vi "WSVCAP SHL FPGA LL Configuration File Handler.vi"(0 "Object Cluster In":T3={"Settings"={"FPGA Resource Name"="", "I2C Slave Address"=20, "I2C Clock Rate (Hz)"=50000.0, "SPI Clock Rate (Hz)"=50000.0, "RFFE Slave Address"=20, "RFFE Clock Rate (Hz)"=50000.0, "Simulate FPGA"=TRUE}, "FPGA Resource"="", "Online"=FALSE, "I2C Wait Ticks"=0, "SPI Wait Ticks"=0, "RFFE Wait Ticks"=0} {"Settings"."RFFE Clock Rate (Hz)" format="%.0f Hz"; "Settings"."RFFE Slave Address" format="0x%02x"; "Settings"."I2C Clock Rate (Hz)" format="%.0f Hz"; "Settings"."SPI Clock Rate (Hz)" format="%.0f Hz"; "Settings"."I2C Slave Address" format="0x%02x"}, 1 "Copy Path":path, 2 "System Cfg":T2={"Configuration File Path"=path "inifiles/System Configuration.ini"}, 7 "Copy Tag":string, 11 "Error In (no error)":errorcluster, 12 "Keys (Empty:All)":T1[](array[typedef]), 13 "Operation":T5) -> (4 "Object Cluster Out":T3={"Settings"={"FPGA Resource Name"="", "I2C Slave Address"=20, "I2C Clock Rate (Hz)"=50000.0, "SPI Clock Rate (Hz)"=50000.0, "RFFE Slave Address"=20, "RFFE Clock Rate (Hz)"=50000.0, "Simulate FPGA"=TRUE}, "FPGA Resource"="", "Online"=FALSE, "I2C Wait Ticks"=0, "SPI Wait Ticks"=0, "RFFE Wait Ticks"=0} {"Settings"."RFFE Clock Rate (Hz)" format="%.0f Hz"; "Settings"."RFFE Slave Address" format="0x%02x"; "Settings"."I2C Clock Rate (Hz)" format="%.0f Hz"; "Settings"."SPI Clock Rate (Hz)" format="%.0f Hz"; "Settings"."I2C Slave Address" format="0x%02x"}, 8 "Cancelled":bool, 15 "Error Out":errorcluster)   [LabVIEW 2012]
uses:
  Type Defs/WSVCAP SHL Core System Cluster.ctl
  Type Defs/WSVCAP SHL I2C Settings Cluster.ctl
  user.lib/Configuration Files/Type Defs/CFG File Operation Enum.ctl
  Type Defs/WSVCAP SHL Configuration Items Enum.ctl
  user.lib/Configuration Files/Type Defs/CFG System Configuration Settings Cluster.ctl
panel:
  in  "Config Enum":T1=enum."Settings::Simulate FPGA"
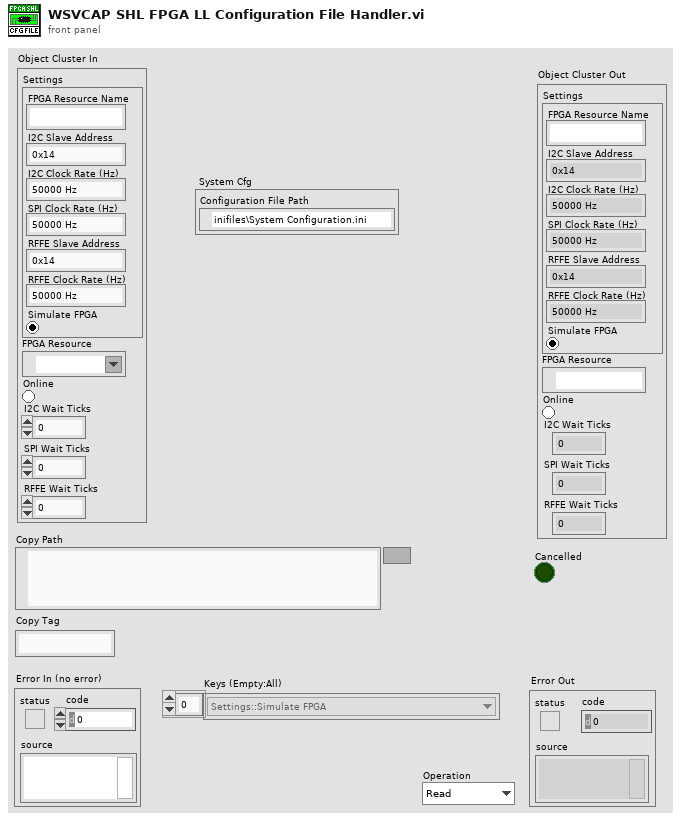
[diagram p1: front panel]
types:
  T1 = typedef "WSVCAP SHL Configuration Items Enum.ctl" = enum16{"Settings::FPGA Resource Name", "Settings::I2C Slave Address", "Settings::I2C Clock Rate (Hz)", "Settings::SPI Clock Rate (Hz)", "Settings::RFFE Slave Address", "Settings::RFFE Clock Rate (Hz)", "Settings::Simulate FPGA"}
  T2 = typedef "CFG System Configuration Settings Cluster.ctl" = cluster{"Configuration File Path":path}
  T3 = typedef "WSVCAP SHL Core System Cluster.ctl" = cluster{"Settings":T4, "FPGA Resource":tag, "Online":bool, "I2C Wait Ticks":u32, "SPI Wait Ticks":u32, "RFFE Wait Ticks":u32}
  T4 = typedef "WSVCAP SHL I2C Settings Cluster.ctl" = cluster{"FPGA Resource Name":string, "I2C Slave Address":u8, "I2C Clock Rate (Hz)":dbl, "SPI Clock Rate (Hz)":dbl, "RFFE Slave Address":u8, "RFFE Clock Rate (Hz)":dbl, "Simulate FPGA":bool}
  T5 = typedef "CFG File Operation Enum.ctl" = enum16{"Read", "Write", "Copy", "Edit"}
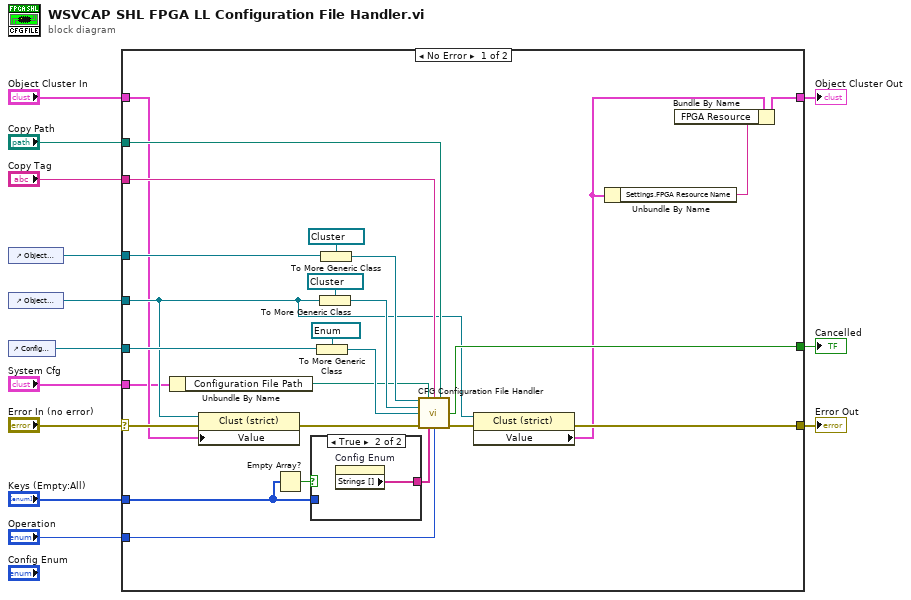
[diagram p0: block diagram]
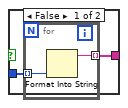
[diagram p2: hidden frame]
diagram:
  n1 = control-ref of="Object Cluster In"() -> (w3:refnum<vi>)
  n2 = control-ref of="Object Cluster Out"() -> (w1:refnum<vi>)
  n3 = control-ref of="Config Enum"() -> (w2:refnum<vi>)
  n4 = case shown="No Error" "Error In (no error)" {
    selector: "Error In (no error)" -> [w22 w46]
    tunnel: [w35 w46] -> w11
    tunnel: "Copy Path" -> [w37 _]
    tunnel: "Copy Tag" -> [w38 _]
    tunnel: "Operation" -> [w39 _]
    tunnel: [w15 w45] -> w7
    tunnel: "Object Cluster In" -> [w19 w45]
    tunnel: w3 -> [w31 _]
    tunnel: w1 -> [w20 _]
    tunnel: w2 -> [w30 _]
    tunnel: "Keys (Empty:All)" -> [w26 _]
    tunnel: [w23 _] -> w5
    tunnel: "System Cfg" -> [w18 _]
    frame No Error {
      n5 = Unbundle By Name(w18) -> ("Configuration File Path"=w17:path)
      n6 = property class="Clust (strict)"(reference=w20, error in=w22, "Value"=w19) -> (error out=w21:errorcluster)  [unwired: 1 out]
      n7 = Empty Array?(array=w26) -> (empty?=w25:bool)
      n8 = case shown="True" w25 {
        tunnel: w26 -> [w41 _]
        tunnel: [w40 w44] -> w24
        frame False {
          n9 = for {
            tunnel: w41 -> [w43] mode=indexing
            tunnel: [w42] -> w40 mode=indexing
            n10 = Format Into String(w43) -> (resulting string=w42:string)  [unwired: 3 in, 1 out]
          }
        }
        frame True {
          n11 = property on="Config Enum" class="Enum (strict)"() -> ("Strings []"=w44:string[])  [unwired: 2 in, 2 out]
        }
      }
      n12 = To More Generic Class(target class=refnum<vi> refnum ("Enum Ref"), reference=w30) -> (generic class reference=w27:refnum<vi>)
      n13 = To More Generic Class(target class=refnum<vi> refnum ("Cluster Ref"), reference=w20) -> (generic class reference=w28:refnum<vi>)
      n14 = To More Generic Class(target class=refnum<vi> refnum ("Cluster Ref"), reference=w31) -> (generic class reference=w29:refnum<vi>)
      n15 = call "CFG Configuration File Handler.vi"("Cluster In Ref"=w29, "System Configuration File"=w17, "Copy Tag"=w38, "Copy Path"=w37, "Cluster Out Ref"=w28, "Enum Ref"=w27, "Error In (no error)"=w21, "Keys (Empty:All)"=w24, "Operation"=w39) -> ("Cancelled"=w23:bool, "Error Out"=w36:errorcluster)  [unwired: 5 in]
      n16 = property class="Clust (strict)"(reference=w20, error in=w36) -> (error out=w35:errorcluster, "Value"=w16:T3)  [unwired: 1 out]
      n17 = Unbundle By Name(w16) -> ("Settings.FPGA Resource Name"=w14:string)
      n18 = Bundle By Name(cluster=w16, "FPGA Resource"=w14) -> (w15:T3)
    }
    frame Error {
    }
  }
  "Object Cluster Out" <- w7
  "Error Out" <- w11
  "Cancelled" <- w5
